vi "rd_actualColumns.vi"(8 "error in (no error)":errorcluster, 11 "Excel refnum":T1) -> (0 "errorout":errorcluster, 3 "Excel refnum out":T1)   [LabVIEW 2017, in "NI_ExcelFile.lvlib"]
uses:
  <vilib>/express/express shared/NI_ExcelFile/NI_ExcelFile.lvlib
  <vilib>/express/express shared/NI_ExcelFile/Ctrls/ExcelRefnum.ctl
  <vilib>/express/express shared/NI_ExcelFile/Ctrls/MainData.ctl
  <vilib>/express/express shared/NI_ExcelFile/Ctrls/StreamMode.ctl
  <vilib>/express/express shared/NI_ExcelFile/Ctrls/TimeColumnMode.ctl
  <vilib>/express/express shared/NI_ExcelFile/Ctrls/FileAttribute.ctl
  <vilib>/express/express shared/NI_ExcelFile/Ctrls/Columns.ctl
  <vilib>/express/express shared/NI_ExcelFile/Ctrls/ColumnInfo.ctl
  <vilib>/express/express shared/NI_ExcelFile/Ctrls/DataType.ctl
  <vilib>/express/express shared/NI_ExcelFile/Ctrls/wd_recordInfo.ctl
  <vilib>/express/express shared/NI_ExcelFile/Ctrls/disk_TemplateFile.ctl
  <vilib>/express/express shared/NI_ExcelFile/Ctrls/meta_file.ctl
  <vilib>/express/express shared/NI_ExcelFile/Ctrls/meta_Block.ctl
  <vilib>/express/express shared/NI_ExcelFile/Ctrls/meta_BlockType.ctl
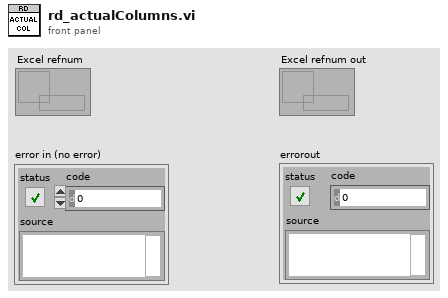
[diagram p1: front panel]
types:
  T1 = typedef "NI_ExcelFile.lvlib/ExcelRefnum.ctl" = refnum<data-value>
  T2 = typedef "NI_ExcelFile.lvlib/MainData.ctl" = cluster{"TargetFile":path, "StreamMode":T3, "Append?":bool, "ChunkSize":u64, "TimeColumnMode":T4, "TimestampFormat":string, "AbsoluteTime?":bool, "FileAttribute ":T5, "Column":T6, "FileRef":refnum<k1>, "MemoryRef":refnum<data-value>[], "RecordInfo":T9[], " ChannelPreviousInfo":u32[], "ChannelFirstRecord":u32[], "PredefinedFormattedValueLength":i64, "DiskTemplate":T10}
  T3 = typedef "NI_ExcelFile.lvlib/StreamMode.ctl" = enum16{"File", "Memory"}
  T4 = typedef "NI_ExcelFile.lvlib/TimeColumnMode.ctl" = enum16{"Empty", "OnePerCh", "One"}
  T5 = typedef "NI_ExcelFile.lvlib/FileAttribute.ctl" = cluster{"Creator":string, "Title":string, "SheetName":string}
  T6 = typedef "NI_ExcelFile.lvlib/Columns.ctl" = T7[]
  T7 = typedef "NI_ExcelFile.lvlib/ColumnInfo.ctl" = cluster{"Header":string, "Format":string, "DataType":T8, "Length":u64}
  T8 = typedef "NI_ExcelFile.lvlib/DataType.ctl" = enum16{"DDT", "WFM", "Array of STR", "Array of DBL", "Array of I8", "Array of I16", "Array of I32", "Array of I64", "Array of SGL", "Array of U8", "Array of U16", "Array of U32", "Array of U64", "Array of Time"}
  T9 = typedef "NI_ExcelFile.lvlib/wd_recordInfo.ctl" = cluster{"ChannelIndex":u32, "StartIndex":u64, "Length":u64, "Previous":i32, "Next":i32}
  T10 = typedef "NI_ExcelFile.lvlib/disk_TemplateFile.ctl" = cluster{"XMLRef":refnum<file>[], "ZipPath":path, "MetaFile":T11, "TempFolder":path}
  T11 = typedef "NI_ExcelFile.lvlib/meta_file.ctl" = cluster{"Ref":refnum<file>, "NextRow":i32, "NextPosition":i64, "Block":T12[]}
  T12 = typedef "NI_ExcelFile.lvlib/meta_Block.ctl" = cluster{"Version":u16, "Type":T13, "Length":i32, "Data":string}
  T13 = typedef "NI_ExcelFile.lvlib/meta_BlockType.ctl" = enum16{"NITag", "File", "Column"}
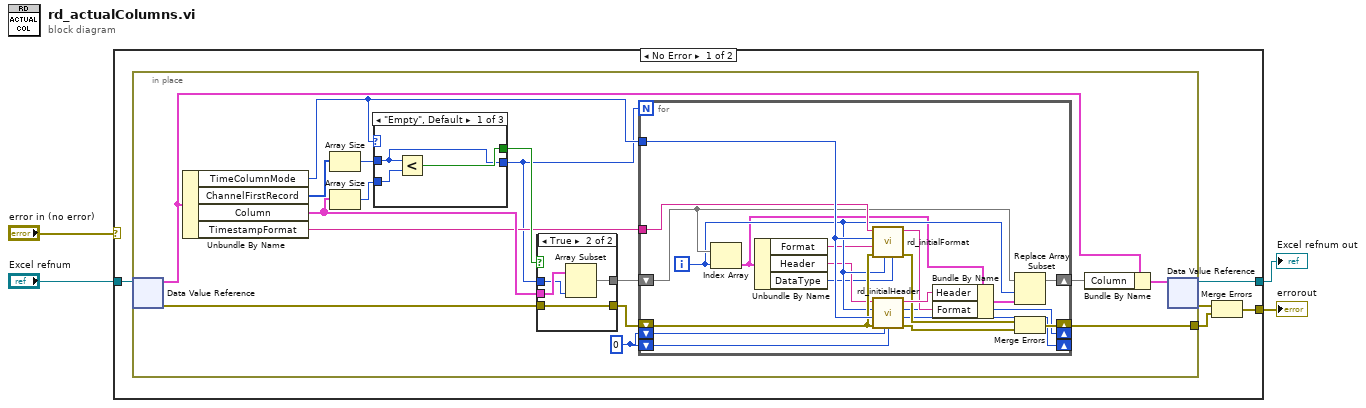
[diagram p0: block diagram]
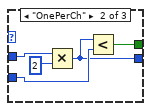
[diagram p3: hidden frame]
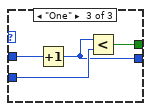
[diagram p4: hidden frame]
diagram:
  n1 = case shown="No Error" "error in (no error)" {
    selector: "error in (no error)" -> [_ w65]
    tunnel: "Excel refnum" -> [w9 w64]
    tunnel: [w8 w64] -> w3
    tunnel: [w6 w65] -> w2
    frame No Error {
      n2 = in-place {
        in-place-border: [w14] -> w5
        w10 = 0
        n3 = in-place-dvr #1(w9) -> (w20:T2, w18:errorcluster)
        n4 = Unbundle By Name(w20) -> ("TimeColumnMode"=w13:T4, "ChannelFirstRecord"=w25:u32[], "Column"=w21:T6, "TimestampFormat"=w12:string)
        n5 = Array Size(array=w25) -> (size(s)=w24:i32)
        n6 = Array Size(array=w21) -> (size(s)=w23:i32)
        n7 = case shown="\"Empty\", Default" w13 {
          tunnel: w24 -> [w52 w58 w62]
          tunnel: w23 -> [w54 w59 w63]
          tunnel: [w53 w56 w61] -> w22
          tunnel: [w52 w55 w60] -> w11
          frame "Empty", Default {
            n8 = Less?(x=w52, y=w54) -> (x < y?=w53:bool)
          }
          frame "OnePerCh" {
            n9 = Multiply(x=w58, y=2) -> (x*y=w55:i32)
            n10 = Less?(x=w55, y=w59) -> (x < y?=w56:bool)
          }
          frame "One" {
            n11 = Increment(x=w62) -> (x+1=w60:i32)
            n12 = Less?(x=w60, y=w63) -> (x < y?=w61:bool)
          }
        }
        n13 = case shown="True" w22 {
          tunnel: [w46 w51] -> w17
          tunnel: w21 -> [w46 w50]
          tunnel: w11 -> [_ w49]
          tunnel: w18 -> [w47 w48]
          tunnel: [w47 w48] -> w16
          frame False {
          }
          frame True {
            n14 = Array Subset(array=w50, length=w49) -> (w51:T6)  [unwired: 1 in]
          }
        }
        n15 = for {
          N: w11 -> [_]
          shift-right: [w39] -> w14
          shift-left: w16 -> [w42]
          tunnel: w13 -> [w43]
          tunnel: w12 -> [w40]
          shift-right: [w37] -> w15
          shift-left: w17 -> [w36]
          shift-right: [w27] -> _
          shift-left: w10 -> [w29]
          shift-right: [w26] -> _
          shift-left: w10 -> [w28]
          i -> [w34]
          n16 = Index Array(array=w36, index=w34) -> (element=w31:T7)
          n17 = Unbundle By Name(w31) -> ("Format"=w33:string, "Header"=w32:string, "DataType"=w30:T8)
          n18 = call <vilib>:"rd_initialFormat.vi"("data type"=w30, "column index"=w34, "error in (no error)"=w42, "column format"=w33, "TimeColumnMode"=w43, "TimestampFormat"=w40) -> ("error out"=w38:errorcluster, "column format out"=w41:string)  [unwired: 4 in]
          n19 = call <vilib>:"rd_initialHeader.vi"("actualTimeIndex"=w28, "actualDataIndex"=w29, "error in (no error)"=w42, "TimeColumnMode"=w43, "column index"=w34, "header"=w32) -> ("error out"=w45:errorcluster, "actualTimeIndex"=w26:i32, "actualDataIndex"=w27:i32, "header out"=w44:string)  [unwired: 2 in]
          n20 = Bundle By Name(cluster=w31, "Header"=w44, "Format"=w41) -> (w35:T7)
          n21 = Replace Array Subset(array=w36, new element=w35, index=w34) -> (w37:T6)
          n22 = Merge Errors(w38, w45) -> (w39:errorcluster)
        }
        n23 = Bundle By Name(cluster=w20, "Column"=w15) -> (w19:T2)
        n24 = in-place-dvr #1(w19) -> (w8:T1, w7:errorcluster)
      }
      n25 = Merge Errors(w7, w5) -> (w6:errorcluster)
    }
    frame Error {
    }
  }
  "Excel refnum out" <- w3
  "errorout" <- w2
